vi "ReadWaveform.vi"(7 "Poll Time (ms)":u32=10, 8 "error in":errorcluster, 9 "Timeout (s)":dbl=5.0, 10 "Samps Read per Chan":i32, 11 "Task in":refnum<class "WaveformTask.lvclass">) -> (0 "error out":errorcluster, 1 "Samples Remaining":u32, 2 "Waveforms":waveform(sgl)[](array[waveform]), 3 "Task out":refnum<class "WaveformTask.lvclass">)   [LabVIEW 2017, in "WaveformTask.lvclass"]
uses:
  WaveformTask.lvclass
  WaveformTask.lvclass/WaveformTask.ctl
  ErrorSelector.ctl
  <vilib>/rvi/errors/niLvFpgaAdjustHostInterfaceError.vi
  <vilib>/Utility/error.llb/Error Cluster From Error Code.vi
  DataFIFOs.ctl
  <vilib>/rvi/interface/nirviMethod/nirviMethod.xnode
  <vilib>/FPGAPlugInAG/Dynamic/niLvFpga_ReadFifo_Dynamic.vi
  <vilib>/rvi/errors/niLvFpgaMergeErrorWithErrorCode.vi
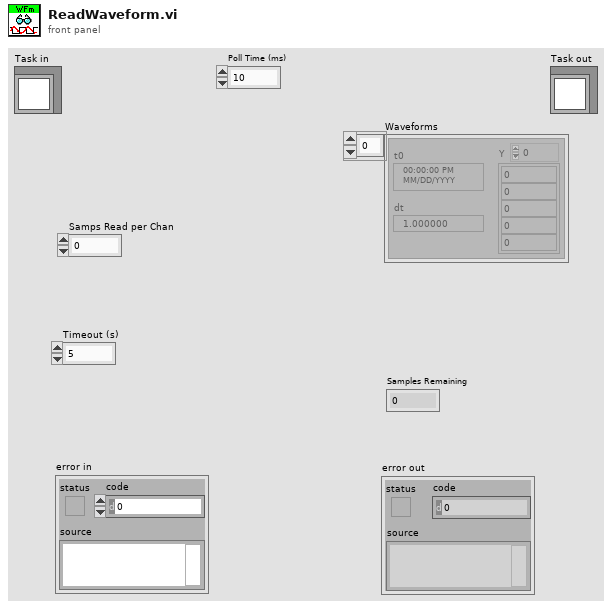
[diagram p1: front panel]
types:
  T1 = typedef "WaveformTask.lvclass/DataFIFOs.ctl" = refnum<k20>
  T2 = typedef "WaveformTask.lvclass/ErrorSelector.ctl" = enum16{"Read Timeout", "Module Underflow", "DMA Overflow", "Chan Count", "Run Timeout", "Start Timeout", "Stop Timeout"}
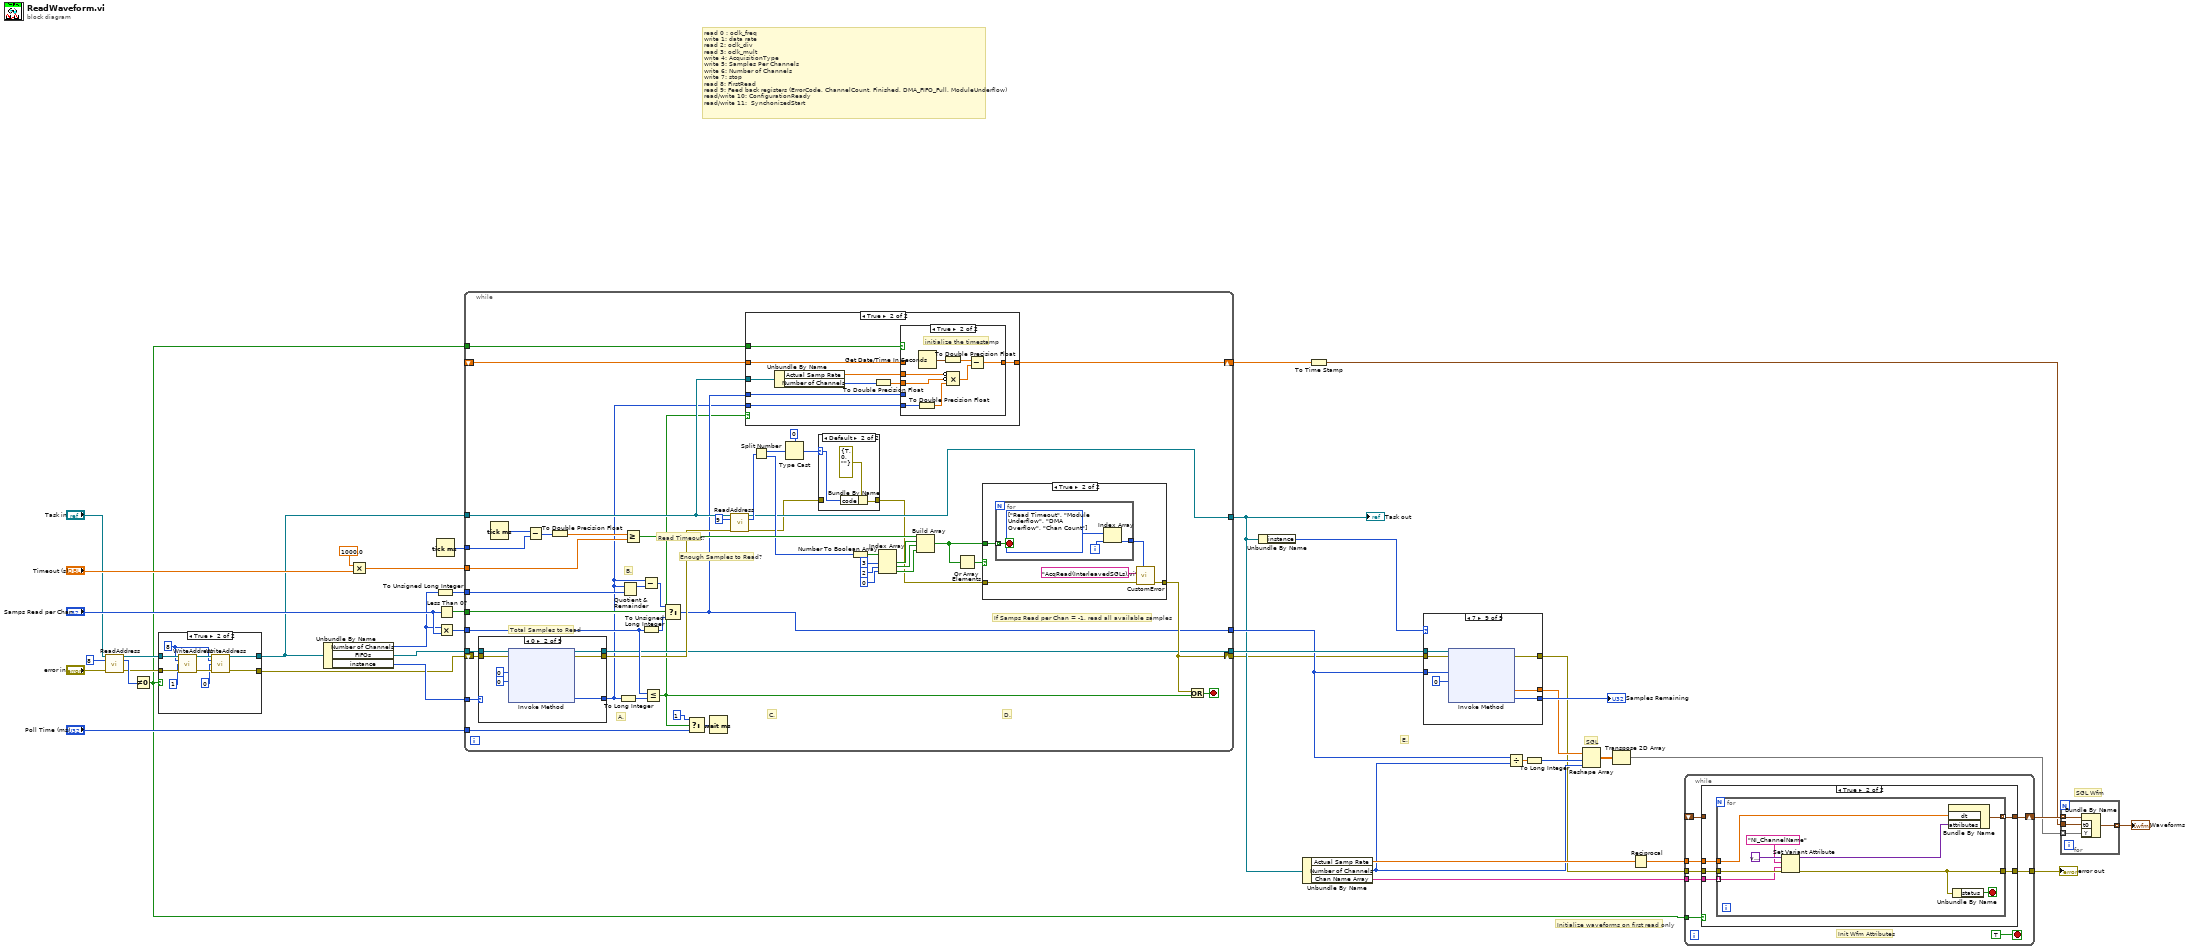
[diagram p0: block diagram]
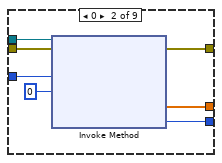
[diagram p5: hidden frame]
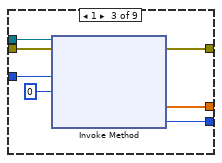
[diagram p6: hidden frame]
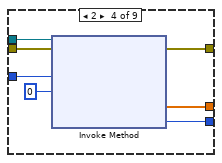
[diagram p7: hidden frame]
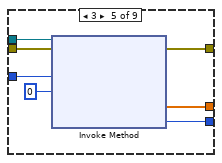
[diagram p8: hidden frame]
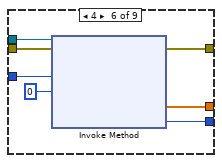
[diagram p9: hidden frame]
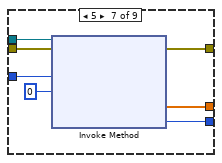
[diagram p10: hidden frame]
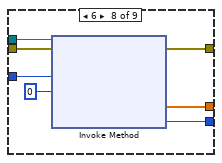
[diagram p11: hidden frame]
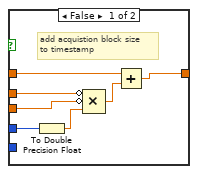
[diagram p13: hidden frame]
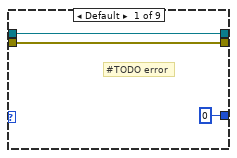
[diagram p15: hidden frame]
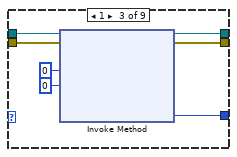
[diagram p16: hidden frame]
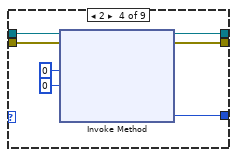
[diagram p17: hidden frame]
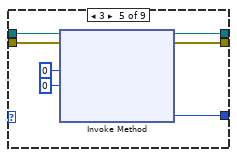
[diagram p18: hidden frame]
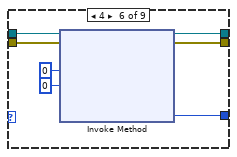
[diagram p19: hidden frame]
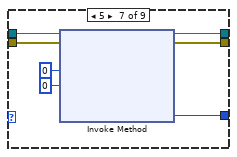
[diagram p20: hidden frame]
diagram:
  # "Initialize waveforms on first read only"
  # "SGL Wfm"
  # "SGL"
  # "read 0 : oclk_freq\nwrite 1: data rate\nread 2: oclk_div\nread 3: oclk_mult\nwrite 4: AcquisitionType\nwrite 5: Samples Per Channels\nwrite 6: Number of Channels\nwrite 7: stop\nread 8: FirstRead\nread 9: Feed back registers (ErrorCode, ChannelCount, Finished, DMA_FIFO_Full, ModuleUnderflow)\nread/write 10: ConfigurationReady\nread/write 11:  SynchonizedStart"
  # "E."
  n1 = call "ReadAddress.vi"("Task in"="Task in", "address"=u64 8, "error in (no error)"="error in") -> ("Task out"=w7:refnum<class "WaveformTask.lvclass">, "data"=w8:u64, "error out"=w6:errorcluster)  [unwired: 10 in]
  n2 = Not Equal To 0?(x=w8) -> (x != 0?=w3:bool)
  n3 = case shown="True" w3 {
    tunnel: w7 -> [w44 w53]
    tunnel: w6 -> [w43 w52]
    tunnel: [w44 w46] -> w5
    tunnel: [w43 w45] -> w4
    frame False {
    }
    frame True {
      w49 = u64 8 ("address")
      n4 = call "WriteAddress.vi"("Task in"=w53, "address"=w49, "data"=u64 1, "error in (no error)"=w52) -> ("Task out"=w51:refnum<class "WaveformTask.lvclass">, "error out"=w50:errorcluster)  [unwired: 10 in]
      n5 = call "WriteAddress.vi"("Task in"=w51, "address"=w49, "data"=u64 0, "error in (no error)"=w50) -> ("Task out"=w46:refnum<class "WaveformTask.lvclass">, "error out"=w45:errorcluster)  [unwired: 10 in]
    }
  }
  n6 = Unbundle By Name(w5) -> ("Number of Channels"=w30:i32, "FIFOs"=w31:T1, "instance"=w29:u8)
  n7 = Multiply(x=1000.0 ("y"), y="Timeout (s)") -> (x*y=w40:dbl)
  n8 = To Unsigned Long Integer(number=w30) -> (unsigned 32bit integer=w36:u32)
  n9 = Tick Count (ms)() -> (millisecond timer value=w42:u32)
  n10 = Less Than 0?(x="Samps Read per Chan") -> (x < 0?=w38:bool)
  n11 = Multiply(x=w30, y="Samps Read per Chan") -> (x*y=w37:i32)
  n12 = while {
    tunnel: [w66] -> w39
    tunnel: w31 -> [w96]
    tunnel: w42 -> [w98]
    tunnel: w40 -> [w97]
    tunnel: "Poll Time (ms)" -> [w91]
    tunnel: [w56] -> w23
    tunnel: w37 -> [w86]
    tunnel: w38 -> [w87]
    tunnel: w36 -> [w88]
    shift-right: [w80] -> w17
    shift-left: w4 -> [w95]
    tunnel: w5 -> [w60]
    tunnel: [w65] -> w19
    tunnel: w29 -> [w64]
    tunnel: w3 -> [w59]
    shift-right: [w58] -> w2
    shift-left: _ -> [w57]
    stop <- w101 stop-if-true
    # "A."
    # "D."
    # "C."
    # "B."
    # "If Samps Read per Chan = -1, read all available samples"
    # "Read Timeout?"
    # "Total Samples to Read"
    # "Enough Samples to Read?"
    n13 = case shown="0" w64 {
      tunnel: w96 -> [w133 w140 w147 w154 w161 w168 w175 w182 w189]
      tunnel: w95 -> [w132 w139 w146 w153 w160 w167 w174 w181 w188]
      tunnel: [u32 0 ("Elements Remaining") w136 w143 w150 w157 w164 w171 w178 w185] -> w54
      tunnel: [w132 w135 w142 w149 w156 w163 w170 w177 w184] -> w73
      tunnel: [w133 w134 w141 w148 w155 w162 w169 w176 w183] -> w66
      frame Default {
        # "#TODO error"
      }
      frame 0 {
        n14 = xnode "Invoke Method"("FPGA VI Reference In"=w140, "error in"=w139, "Number of Elements"=u32 0, "Timeout (ms)"=0) -> ("FPGA VI Reference Out"=w134:T1, "error out"=w135:errorcluster, "Elements Remaining"=w136:u32)  [unwired: 1 out]
      }
      frame 1 {
        n15 = xnode "Invoke Method"("FPGA VI Reference In"=w147, "error in"=w146, "Number of Elements"=u32 0, "Timeout (ms)"=0) -> ("FPGA VI Reference Out"=w141:T1, "error out"=w142:errorcluster, "Elements Remaining"=w143:u32)  [unwired: 1 out]
      }
      frame 2 {
        n16 = xnode "Invoke Method"("FPGA VI Reference In"=w154, "error in"=w153, "Number of Elements"=u32 0, "Timeout (ms)"=0) -> ("FPGA VI Reference Out"=w148:T1, "error out"=w149:errorcluster, "Elements Remaining"=w150:u32)  [unwired: 1 out]
      }
      frame 3 {
        n17 = xnode "Invoke Method"("FPGA VI Reference In"=w161, "error in"=w160, "Number of Elements"=u32 0, "Timeout (ms)"=0) -> ("FPGA VI Reference Out"=w155:T1, "error out"=w156:errorcluster, "Elements Remaining"=w157:u32)  [unwired: 1 out]
      }
      frame 4 {
        n18 = xnode "Invoke Method"("FPGA VI Reference In"=w168, "error in"=w167, "Number of Elements"=u32 0, "Timeout (ms)"=0) -> ("FPGA VI Reference Out"=w162:T1, "error out"=w163:errorcluster, "Elements Remaining"=w164:u32)  [unwired: 1 out]
      }
      frame 5 {
        n19 = xnode "Invoke Method"("FPGA VI Reference In"=w175, "error in"=w174, "Number of Elements"=u32 0, "Timeout (ms)"=0) -> ("FPGA VI Reference Out"=w169:T1, "error out"=w170:errorcluster, "Elements Remaining"=w171:u32)  [unwired: 1 out]
      }
      frame 6 {
        n20 = xnode "Invoke Method"("FPGA VI Reference In"=w182, "error in"=w181, "Number of Elements"=u32 0, "Timeout (ms)"=0) -> ("FPGA VI Reference Out"=w176:T1, "error out"=w177:errorcluster, "Elements Remaining"=w178:u32)  [unwired: 1 out]
      }
      frame 7 {
        n21 = xnode "Invoke Method"("FPGA VI Reference In"=w189, "error in"=w188, "Number of Elements"=u32 0, "Timeout (ms)"=0) -> ("FPGA VI Reference Out"=w183:T1, "error out"=w184:errorcluster, "Elements Remaining"=w185:u32)  [unwired: 1 out]
      }
    }
    n22 = Tick Count (ms)() -> (millisecond timer value=w94:u32)
    n23 = Subtract(x=w94, y=w98) -> (x-y=w100:u32)
    n24 = To Double Precision Float(number=w100) -> (double precision float=w99:dbl)
    n25 = To Long Integer(number=w54) -> (32bit integer=w89:i32)
    n26 = Quotient & Remainder(x=w54, y=w88) -> (x-y*floor(x/y)=w84:u32)  [unwired: 1 out]
    n27 = Greater Or Equal?(x=w99, y=w97) -> (x >= y?=w93:bool)
    n28 = Subtract(x=w54, y=w84) -> (x-y=w83:u32)
    n29 = To Unsigned Long Integer(number=w86) -> (unsigned 32bit integer=w85:u32)
    n30 = Less Or Equal?(x=w86, y=w89) -> (x <= y?=w55:bool)
    n31 = Select(t=w83, s=w87, f=w85) -> (s? t:f=w56:u32)
    n32 = Select(t=u32 1, s=w55, f=w91) -> (s? t:f=w92:u32)
    n33 = Wait (ms)(milliseconds to wait=w92) -> ()  [unwired: 1 out]
    n34 = call "ReadAddress.vi"("Task in"=w60, "address"=u64 9, "error in (no error)"=w73) -> ("Task out"=w65:refnum<class "WaveformTask.lvclass">, "data"=w78:u64, "error out"=w62:errorcluster)  [unwired: 10 in]
    n35 = case shown="True" w55 {
      tunnel: w57 -> [w102 w111]
      tunnel: w59 -> [_ w110]
      tunnel: w60 -> [_ w108]
      tunnel: w54 -> [_ w107]
      tunnel: [w102 w106] -> w58
      tunnel: w56 -> [_ w105]
      frame False {
      }
      frame True {
        n36 = Unbundle By Name(w108) -> ("Actual Samp Rate"=w109:dbl, "Number of Channels"=w104:i32)
        n37 = To Double Precision Float(number=w104) -> (double precision float=w103:dbl)
        n38 = case shown="True" w110 {
          tunnel: w109 -> [w116 w126]
          tunnel: w111 -> [w117 _]
          tunnel: w105 -> [w113 _]
          tunnel: w103 -> [w114 w125]
          tunnel: w107 -> [_ w120]
          tunnel: [w118 w122] -> w106
          frame False {
            # "add acquistion block size\nto timestamp"
            n39 = To Double Precision Float(number=w113) -> (double precision float=w112:dbl)
            n40 = Compound Arithmetic op=MULTIPLY(invert w116, invert w114, w112) -> (w115:dbl)
            n41 = Add(x=w117, y=w115) -> (x+y=w118:dbl)
          }
          frame True {
            # "initialize the timestamp"
            n42 = To Double Precision Float(number=w120) -> (double precision float=w119:dbl)
            n43 = Get Date/Time In Seconds() -> (seconds since 1Jan1904=w124:timestamp)
            n44 = To Double Precision Float(number=w124) -> (double precision float=w121:dbl)
            n45 = Compound Arithmetic op=MULTIPLY(invert w126, invert w125, w119) -> (w123:dbl)
            n46 = Subtract(x=w121, y=w123) -> (x-y=w122:dbl)
          }
        }
      }
    }
    n47 = Split Number(x=w78) -> (hi(x)=w77:u32, lo(x)=w75:u32)
    n48 = Type Cast(type=0, x=w77) -> (*(type *) &x=w63:i32)
    n49 = case shown="Default" w63 {
      selector: w63 -> [_ w129]
      tunnel: w62 -> [w127 _]
      tunnel: [w127 w128] -> w61
      frame 0 {
      }
      frame Default {
        n50 = Bundle By Name(cluster=errorcluster {"status"=TRUE, "code"=0, "source"=""} ("error out"), "code"=w129) -> (w128:errorcluster)
      }
    }
    n51 = Number To Boolean Array(number=w75) -> (Boolean array=w74:bool[])
    n52 = Index Array(array=w74, index #1=3 ("index"), index #2=2 ("index"), index #3=0 ("index")) -> (element #1=w69:bool, element #2=w68:bool, element #3=w67:bool)
    n53 = Build Array(w93, w69, w68, w67) -> (w81:bool[])
    n54 = Or Array Elements(Boolean array=w81) -> (logical OR=w82:bool)
    n55 = case shown="True" w82 {
      tunnel: [w190 w194] -> w80
      tunnel: w61 -> [w190 w195]
      tunnel: w81 -> [_ w193]
      frame False {
      }
      frame True {
        n56 = for {
          tunnel: w193 -> [w199] mode=indexing
          tunnel: [w197] -> w192
          i -> [w198]
          stop <- w199 stop-if-true
          w196 = T2[] [enum."Read Timeout", enum."Module Underflow", enum."DMA Overflow", enum."Chan Count"] items=["Read Timeout", "Module Underflow", "DMA Overflow", "Chan Count", "Run Timeout", "Start Timeout", "Stop Timeout"]
          n57 = Index Array(array=w196, index=w198) -> (element=w197:T2)
        }
        n58 = call "CustomError.vi"("Error Selector"=w192, "error in (no error)"=w195, "VI name"="AcqRead(InterleavedSGLs).vi" ("Calling VI")) -> ("error out"=w194:errorcluster)  [unwired: 8 in]
      }
    }
    n59 = Or(x=w80, y=w55) -> (x .or. y?=w101:bool)
  }
  "Task out" <- w19
  n60 = Unbundle By Name(w19) -> ("instance"=w28:u8)
  n61 = Unbundle By Name(w19) -> ("Actual Samp Rate"=w22:dbl, "Number of Channels"=w18:i32, "Chan Name Array"=w1:string[])
  n62 = To Time Stamp(1:w2) -> (0:w13:timestamp)
  n63 = case shown="7" w28 {
    tunnel: [w200 w207 w214 w221 w228 w235 w242 w249 w256] -> w16
    tunnel: w17 -> [w200 w206 w213 w220 w227 w234 w241 w248 w255]
    tunnel: w39 -> [_ w205 w212 w219 w226 w233 w240 w247 w254]
    tunnel: w23 -> [_ w204 w211 w218 w225 w232 w239 w246 w253]
    tunnel: [_ w202 w209 w216 w223 w230 w237 w244 w251] -> w24
    tunnel: [_ w201 w208 w215 w222 w229 w236 w243 w250] -> w32
    frame Default {
      # "#TODO Error"
    }
    frame 0 {
      n64 = xnode "Invoke Method"("FPGA VI Reference In"=w205, "error in"=w206, "Number of Elements"=w204, "Timeout (ms)"=0) -> ("error out"=w207:errorcluster, "Data"=w202:sgl[], "Elements Remaining"=w201:u32)  [unwired: 1 out]
    }
    frame 1 {
      n65 = xnode "Invoke Method"("FPGA VI Reference In"=w212, "error in"=w213, "Number of Elements"=w211, "Timeout (ms)"=0) -> ("error out"=w214:errorcluster, "Data"=w209:sgl[], "Elements Remaining"=w208:u32)  [unwired: 1 out]
    }
    frame 2 {
      n66 = xnode "Invoke Method"("FPGA VI Reference In"=w219, "error in"=w220, "Number of Elements"=w218, "Timeout (ms)"=0) -> ("error out"=w221:errorcluster, "Data"=w216:sgl[], "Elements Remaining"=w215:u32)  [unwired: 1 out]
    }
    frame 3 {
      n67 = xnode "Invoke Method"("FPGA VI Reference In"=w226, "error in"=w227, "Number of Elements"=w225, "Timeout (ms)"=0) -> ("error out"=w228:errorcluster, "Data"=w223:sgl[], "Elements Remaining"=w222:u32)  [unwired: 1 out]
    }
    frame 4 {
      n68 = xnode "Invoke Method"("FPGA VI Reference In"=w233, "error in"=w234, "Number of Elements"=w232, "Timeout (ms)"=0) -> ("error out"=w235:errorcluster, "Data"=w230:sgl[], "Elements Remaining"=w229:u32)  [unwired: 1 out]
    }
    frame 5 {
      n69 = xnode "Invoke Method"("FPGA VI Reference In"=w240, "error in"=w241, "Number of Elements"=w239, "Timeout (ms)"=0) -> ("error out"=w242:errorcluster, "Data"=w237:sgl[], "Elements Remaining"=w236:u32)  [unwired: 1 out]
    }
    frame 6 {
      n70 = xnode "Invoke Method"("FPGA VI Reference In"=w247, "error in"=w248, "Number of Elements"=w246, "Timeout (ms)"=0) -> ("error out"=w249:errorcluster, "Data"=w244:sgl[], "Elements Remaining"=w243:u32)  [unwired: 1 out]
    }
    frame 7 {
      n71 = xnode "Invoke Method"("FPGA VI Reference In"=w254, "error in"=w255, "Number of Elements"=w253, "Timeout (ms)"=0) -> ("error out"=w256:errorcluster, "Data"=w251:sgl[], "Elements Remaining"=w250:u32)  [unwired: 1 out]
    }
  }
  "Samples Remaining" <- w32
  n72 = Divide(x=w23, y=w18) -> (x/y=w26:dbl)
  n73 = To Long Integer(number=w26) -> (32bit integer=w25:i32)
  n74 = Reshape Array(w24, w25, w18) -> (w27:sgl[][])
  n75 = Transpose 2D Array(2D array=w27) -> (transposed array=w15:sgl[][])
  n76 = Reciprocal(x=w22) -> (1/x=w21:dbl)
  n77 = while {
    tunnel: w21 -> [w264]
    tunnel: w16 -> [w263]
    tunnel: [w262] -> w14
    tunnel: w1 -> [w261]
    shift-right: [w260] -> w20
    shift-left: _ -> [w258]
    tunnel: w3 -> [w257]
    stop <- TRUE stop-if-true
    # "Init Wfm Attributes"
    n78 = case shown="True" w257 {
      tunnel: w264 -> [_ w271]
      tunnel: w263 -> [w266 w270]
      tunnel: [w266 w269] -> w262
      tunnel: w261 -> [_ w268]
      tunnel: [w265 w267] -> w260
      tunnel: w258 -> [w265 _]
      frame False {
      }
      frame True {
        n79 = for {
          tunnel: w271 -> [w280]
          tunnel: [w279] -> w267 mode=indexing
          tunnel: w270 -> [w278]
          tunnel: [w272] -> w269
          tunnel: w268 -> [w274] mode=indexing
          stop <- w277 stop-if-true
          n80 = Set Variant Attribute(Variant=variant ("variant out"), name="NI_ChannelName", value=w274, error in=w278) -> (Variant out=w273:variant, error out=w272:errorcluster)  [unwired: 1 out]
          n81 = Bundle By Name("dt"=w280, "attributes"=w273) -> (w279:waveform(sgl))  [unwired: 1 out]
          n82 = Unbundle By Name(w272) -> ("status"=w277:bool)
        }
      }
    }
  }
  "error out" <- w14
  n83 = for {
    tunnel: w20 -> [w284] mode=indexing
    tunnel: w13 -> [w283]
    tunnel: [w282] -> w12 mode=indexing
    tunnel: w15 -> [w281] mode=indexing
    n84 = Bundle By Name(cluster=w284, "t0"=w283, "Y"=w281) -> (w282:waveform(sgl))
  }
  "Waveforms" <- w12
